vi "InterTrial.vi"(8 "error in (no error)":errorcluster, 11 "TrialBasedExperiment in":refnum<class "MatlabExperiment.lvclass">) -> (0 "error out":errorcluster, 2 "Timeout":dbl, 3 "TrialBasedExperiment out":refnum<class "MatlabExperiment.lvclass">)   [LabVIEW 2014, in "AcquisitionCoreObjects.lvlib" / "MatlabExperiment.lvclass"]
uses:
  MatlabExperiment.lvclass
  TrialBasedExperimentObject/TrialBasedExperiment.lvclass
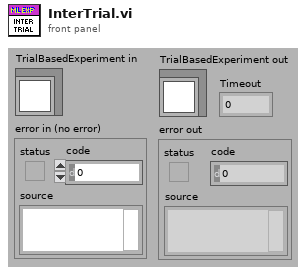
[diagram p1: front panel]
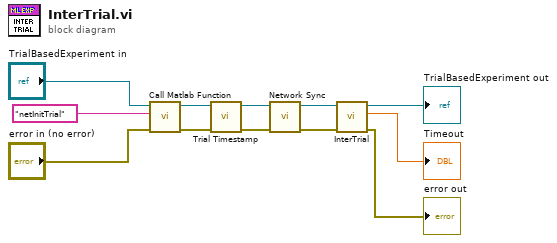
[diagram p0: block diagram]
diagram:
  n1 = call-dynamic "Call Matlab Function.vi"("error in (no error)"="error in (no error)", "Function name"="netInitTrial", "TrialBasedExperiment in"="TrialBasedExperiment in") -> ("error out"=w3:errorcluster, "TrialBasedExperiment out"=w4:refnum<class "MatlabExperiment.lvclass">)  [unwired: 5 in, 2 out]
  n2 = call-dynamic "Trial Timestamp.vi"("error in (no error)"=w3, "TrialBasedExperiment in"=w4) -> ("error out"=w1:errorcluster, "TrialBasedExperiment out"=w2:refnum<class "MatlabExperiment.lvclass">)  [unwired: 8 in]
  n3 = call "Network Sync.vi"("error in (no error)"=w1, "MatlabExperiment in"=w2) -> ("error out"=w6:errorcluster, "MatlabExperiment out"=w5:refnum<class "MatlabExperiment.lvclass">)  [unwired: 8 in]
  n4 = call-parent "InterTrial.vi"("error in (no error)"=w6, "TrialBasedExperiment in"=w5) -> ("error out"=→"error out":errorcluster, "Timeout"=→"Timeout":dbl, "TrialBasedExperiment out"=→"TrialBasedExperiment out":refnum<class "MatlabExperiment.lvclass">)  [unwired: 7 in]
